vi "veristandSteps-typePaletteFile-update.vi"() -> ()   [LabVIEW 2014, in "veristand-steps-build-system.lvlib"]
uses:
  <vilib>/xml/Load XML File.vi
  <vilib>/xml/Close Reference(Node).vi
  <vilib>/xml/Close Reference(NNMap).vi
  veristand-steps-build-system.lvlib
  <resource>/objmgr/DOMUserDefRef.rc
  <vilib>/xml/NI_XML.lvlib
  <vilib>/ni/Simple XML/Simple XML.lvlib
  <vilib>/Wiresmith Technology/LabVIEW CLI/CLI Class/CLI.lvclass
panel:
  out "error out":errorcluster
  # "Arguments\n1: Old TS ini File Location\n2: New TS ini File Location\n3: New VS Assembly Version\n4: New Steps Version String\n5: New VS InstallPath"
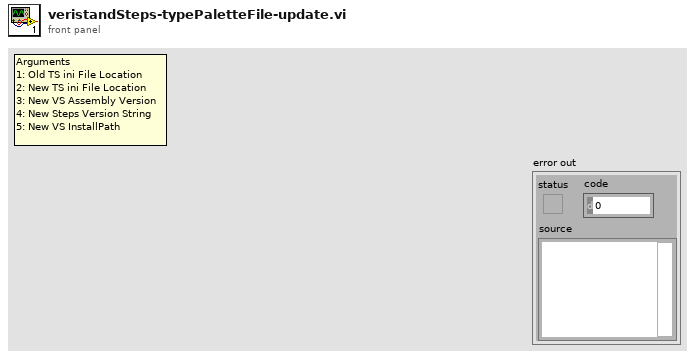
[diagram p1: front panel]
types:
  T1 = enum32{"invalid app kind", "Development System", "Run Time System", "Student Edition", "Embedded LabVIEW", "Evaluation", "Custom"}
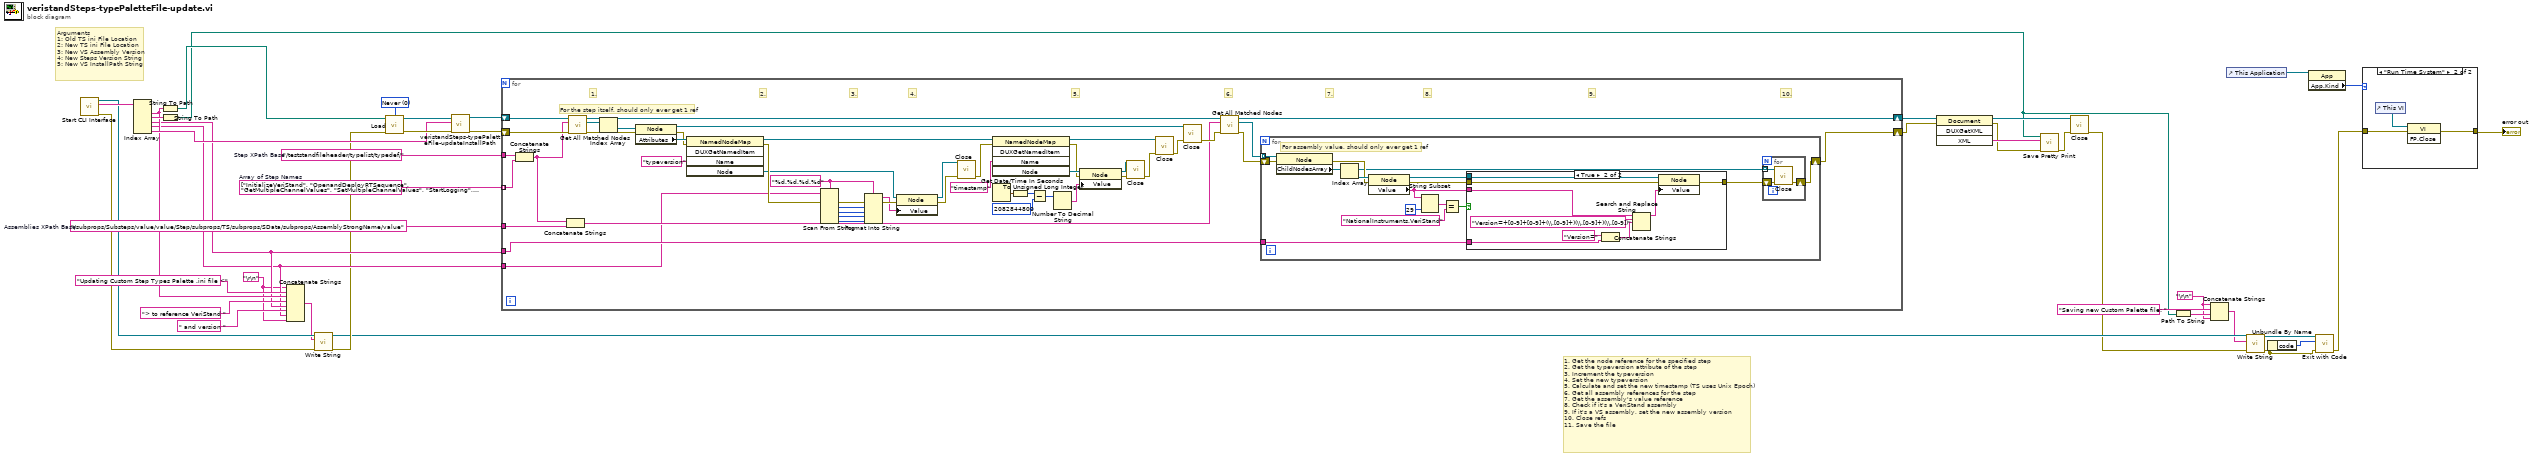
[diagram p0: block diagram]
diagram:
  w6 = "\r\n"
  w14 = "\r\n"
  w26 = "/subprops/Substeps/value/value/Step/subprops/TS/subprops/SData/subprops/AssemblyStrongName/value"  # Assemblies XPath Base
  w36 = string[] ["InitializeVeriStand", "OpenandDeployRTSequence", "GetMultipleChannelValues", "SetMultipleChannelValues", "StartLogging", "StopLogging", "StopVeriStand", "RunProject", "ConnectProject", "DisconnectProject", "UndeployProject", "RunStimulusProfileAsynch", "DeployProject", "OpenReferences", "GetAlarmState", "SetChannelValue", "GetAlarmList", "RunStimulusProfileBlocking", "SetAlarmState", "SetModelParameterValue", "CloseProject", "UpdateModelParametersFromFile", "GetChannelValue", "LimitTestChannelValue", "GetChannelFaultValue", "GetModelParameterValue", "ClearFault", "ClearAllFaults", "PauseRTSequence", "StopRTSequence", "GetSequenceState", "GetAllSequenceNames", "StartRTSequence", "AbortRTSequence", "GetSequenceReturnValue", "StartStimulusProfileSession", "RunRTSequenceAction", "CloseWorkspace", "OpenWorkspace", "SilentConnect", "SilentDisconnect", "OpenProject", "RunRTSequencePassFail", "RunRTSequenceNumericLimit", "SetChannelFaultValue", "StopVeristandGateway", "StartVeristand"]  # Array of Step Names
  w42 = "/teststandfileheader/typelist/typedef/"  # Step XPath Base
  w43 = 0 items=["Never", "Always", "Auto"] ("validate on load (Auto)")
  # "Arguments\n1: Old TS ini File Location\n2: New TS ini File Location\n3: New VS Assembly Version\n4: New Steps Version String\n5: New VS InstallPath String"
  # "1. Get the node reference for the specified step\n2. Get the typeversion attribute of the step\n3. Increment the typeversion\n4. Set the new typeversion\n5. Calculate and set the new timestamp (TS uses Unix Epoch)\n6. Get all assembly references for the step\n7. Get the assembly's value reference\n8. Check if it's a VeriStand assembly\n9. If it's a VS assembly, set the new assembly version\n10. Close refs\n11. Save the file"
  n1 = call <vilib>:"Start CLI Interface.vi"() -> ("error out"=w22:errorcluster, "Custom Parameters"=w23:string[], "CLI out"=w21:refnum<class "CLI.lvclass">)  [unwired: 9 in]
  n2 = Index Array(array=w23) -> (element #1=w19:string, element #2=w24:string, element #3=w17:string, element #4=w15:string, element #5=w25:string)  [unwired: 5 in]
  n3 = String To Path(string=w19) -> (path=w35:path)
  n4 = String To Path(string=w24) -> (path=w8:path)
  n5 = Concatenate Strings(w14, "Updating Custom Step Types Palette .ini file <", w19, "> to reference VeriStand " ("string"), w17, " and version " ("string"), w15, w14) -> (w13:string)
  n6 = call <vilib>:"Write String.vi"("error in (no error)"=w22, "Text to Write"=w13, "CLI in"=w21) -> ("error out"=w12:errorcluster, "CLI out"=w11:refnum<class "CLI.lvclass">)  [unwired: 7 in]
  n7 = call-poly <vilib>:"Load.vi"("path to XML document"=w35, "validate on load (Auto)"=w43, "error in (no error)"=w12) -> ("DOM document out"=w30:refnum<k20>, "error out"=w31:errorcluster)  [unwired: 10 in, 1 out]
  n8 = call "veristandSteps-typePaletteFile-updateInstallPath.vi"("error in (no error)"=w31, "New VS InstallPath"=w25, "DOM document in"=w30) -> ("error out"=w29:errorcluster, "DOM document out"=w28:refnum<k20>)  [unwired: 7 in]
  n9 = for {
    tunnel: w36 -> [w89] mode=indexing
    shift-right: [w87] -> w41
    shift-left: w28 -> [w92]
    tunnel: w42 -> [w90]
    shift-right: [w80] -> w27
    shift-left: w29 -> [w91]
    tunnel: w26 -> [w85]
    tunnel: w17 -> [w48]
    tunnel: w15 -> [w45]
    w69 = "%d.%d.%d.%d" ("format string")
    # "10."
    # "9."
    # "8."
    # "7."
    # "6."
    # "5."
    # "4."
    # "3."
    # "2."
    # "1."
    # "For the step itself, should only ever get 1 ref"
    n10 = Concatenate Strings(w90, w89) -> (w84:string)
    n11 = Concatenate Strings(w84, w85) -> (w83:string)
    n12 = call <vilib>:"Get All Matched Nodes.vi"("error in (no error)"=w91, "XPath expression"=w84, "node in"=w92) -> ("error out"=w75:errorcluster, "node result array"=w79:refnum<k20>[], "node out"=w88:refnum<k20>)  [unwired: 6 in]
    n13 = Index Array(array=w79) -> (element=w78:refnum<k20>)  [unwired: 1 in]
    n14 = property class="Node"(reference=w78, error in=w75) -> (reference out=w53:refnum<k20>, error out=w76:errorcluster, "Attributes"=w77:refnum<k20>)
    n15 = invoke class="NamedNodeMap" method="DUXGetNamedItem"(reference=w77, error in=w76, "Name"="typeversion") -> (reference out=w68:refnum<k20>, error out=w46:errorcluster, "Node"=w44:refnum<k20>)  [unwired: 2 in, 2 out]
    n16 = Scan From String(format string=w69, input string=w45, error in=w46) -> (error out=w73:errorcluster, output 1=w72:i32, output 2=w71:i32, output 3=w70:i32, output 4=w47:i32)  [unwired: 5 in, 2 out]
    n17 = Format Into String(format string=w69, error in=w73, w72, w71, w70, w47) -> (resulting string=w66:string, error out=w67:errorcluster)  [unwired: 1 in]
    n18 = property class="Node"(reference=w44, error in=w67, "Value"=w66) -> (reference out=w64:refnum<k20>, error out=w65:errorcluster)
    n19 = call-poly <vilib>:"Close.vi"("error in (no error)"=w65, "node"=w64) -> ("error out"=w63:errorcluster)  [unwired: 7 in]
    n20 = invoke class="NamedNodeMap" method="DUXGetNamedItem"(reference=w68, error in=w63, "Name"="timestamp") -> (reference out=w56:refnum<k20>, error out=w60:errorcluster, "Node"=w61:refnum<k20>)  [unwired: 2 in, 2 out]
    n21 = Get Date/Time In Seconds() -> (seconds since 1Jan1904=w52:timestamp)
    n22 = To Unsigned Long Integer(number=w52) -> (unsigned 32bit integer=w51:u32)
    n23 = Subtract(x=w51, y=u32 2082844800) -> (x-y=w49:u32)
    n24 = Number To Decimal String(number=w49) -> (decimal integer string=w59:string)  [unwired: 1 in]
    n25 = property class="Node"(reference=w61, error in=w60, "Value"=w59) -> (reference out=w57:refnum<k20>, error out=w58:errorcluster)
    n26 = call-poly <vilib>:"Close.vi"("error in (no error)"=w58, "node"=w57) -> ("error out"=w55:errorcluster)  [unwired: 7 in]
    n27 = call-poly <vilib>:"Close.vi"("error in (no error)"=w55, "named node map"=w56) -> ("error out"=w54:errorcluster)  [unwired: 7 in]
    n28 = call-poly <vilib>:"Close.vi"("error in (no error)"=w54, "node"=w53) -> ("error out"=w86:errorcluster)  [unwired: 7 in]
    n29 = call <vilib>:"Get All Matched Nodes.vi"("error in (no error)"=w86, "XPath expression"=w83, "node in"=w88) -> ("error out"=w81:errorcluster, "node result array"=w82:refnum<k20>[], "node out"=w87:refnum<k20>)  [unwired: 6 in]
    n30 = for {
      tunnel: w82 -> [w107] mode=indexing
      shift-right: [w102] -> w80
      shift-left: w81 -> [w106]
      tunnel: w48 -> [w93]
      # "For assembly value, should only ever get 1 ref"
      n31 = property class="Node"(reference=w107, error in=w106) -> (error out=w104:errorcluster, "ChildNodesArray"=w103:refnum<k20>[])  [unwired: 1 out]
      n32 = Index Array(array=w103) -> (element=w105:refnum<k20>)  [unwired: 1 in]
      n33 = property class="Node"(reference=w105, error in=w104) -> (reference out=w99:refnum<k20>, error out=w100:errorcluster, "Value"=w98:string)
      n34 = String Subset(string=w98, length (rest)=29 ("length (rest)")) -> (substring=w96:string)  [unwired: 1 in]
      n35 = Equal?(x=w96, y="NationalInstruments.VeriStand" ("Node Value 2")) -> (x = y?=w94:bool)
      n36 = case shown="True" w94 {
        tunnel: w98 -> [_ w117]
        tunnel: [w108 w113] -> w101
        tunnel: w100 -> [w108 w111]
        tunnel: w99 -> [_ w110]
        tunnel: w93 -> [_ w109]
        frame False {
        }
        frame True {
          n37 = Concatenate Strings("Version=" ("replace string (\"\")"), w109) -> (w114:string)
          n38 = Search and Replace String(input string=w117, search string="Version=+[0-9]+[0-9]+(\\.[0-9]+)(\\.[0-9]+)(\\.[0-9])", replace string=w114) -> (result string=w112:string)  [unwired: 5 in, 3 out]
          n39 = property class="Node"(reference=w110, error in=w111, "Value"=w112) -> (error out=w113:errorcluster)  [unwired: 1 out]
        }
      }
      n40 = for {
        tunnel: w103 -> [w120] mode=indexing
        shift-right: [w118] -> w102
        shift-left: w101 -> [w119]
        n41 = call-poly <vilib>:"Close.vi"("error in (no error)"=w119, "node"=w120) -> ("error out"=w118:errorcluster)  [unwired: 7 in]
      }
    }
  }
  n42 = invoke class="Document" method="DUXGetXML"(reference=w41, error in=w27) -> (reference out=w38:refnum<k20>, error out=w39:errorcluster, "XML"=w40:string)  [unwired: 2 in, 1 out]
  n43 = call <vilib>:"Save Pretty Print.vi"("error in (no error)"=w39, "Pretty XML String"=w40, "XML file path"=w8) -> ("error out"=w37:errorcluster)  [unwired: 7 in, 1 out]
  n44 = call-poly <vilib>:"Close.vi"("error in (no error)"=w37, "node"=w38) -> ("error out"=w10:errorcluster)  [unwired: 7 in]
  n45 = Path To String(path=w8) -> (string=w7:string)
  n46 = Concatenate Strings(w6, "Saving new Custom Palette file: ", w7, w6) -> (w5:string)
  n47 = control-ref of="This Application"() -> (w34:refnum<vi>)
  n48 = call <vilib>:"Write String.vi"("error in (no error)"=w10, "Text to Write"=w5, "CLI in"=w11) -> ("error out"=w2:errorcluster, "CLI out"=w4:refnum<class "CLI.lvclass">)  [unwired: 7 in]
  n49 = Unbundle By Name(w2) -> ("code"=w3:i32)
  n50 = property class="App"(reference=w34) -> ("App.Kind"=w33:T1)  [unwired: 1 in, 2 out]
  n51 = call <vilib>:"Exit with Code.vi"("error in (no error)"=w2, "Exit Code (0)"=w3, "CLI in"=w4) -> ("error out"=w1:errorcluster)  [unwired: 8 in]
  n52 = case shown="\"Run Time System\"" w33 {
    tunnel: w1 -> [w121 w123]
    tunnel: [w121 w122] -> w32
    frame "Development System", Default {
    }
    frame "Run Time System" {
      n53 = control-ref of="This VI"() -> (w124:refnum<vi>)
      n54 = invoke class="VI" method="FP.Close"(reference=w124, error in=w123) -> (error out=w122:errorcluster)  [unwired: 1 in, 2 out]
    }
  }
  "error out" <- w32
